vi "Write Case Sensitive Pop-up.vi"(8 "error in (no error)":errorcluster, 10 "CaseSensitivePopup":bool, 11 "ComboBox.lvclass in":refnum<class "ComboBox.lvclass">) -> (0 "error out":errorcluster, 3 "ComboBox.lvclass out":refnum<class "ComboBox.lvclass">)   [LabVIEW 2015, in "ComboBox.lvclass"]
uses:
  ComboBox.lvclass
  ComboBox.lvclass/ComboBox.ctl
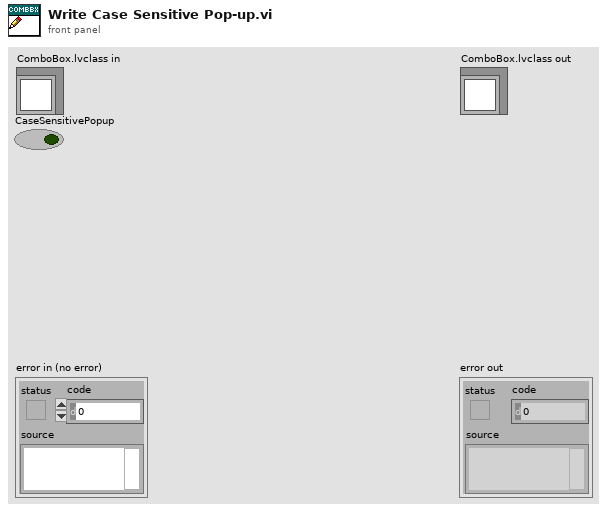
[diagram p1: front panel]
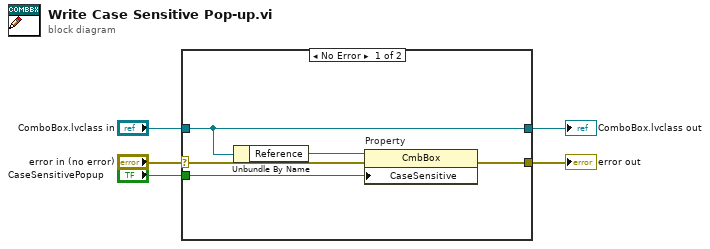
[diagram p0: block diagram]
diagram:
  n1 = case shown="No Error" "error in (no error)" {
    selector: "error in (no error)" -> [w6 w12]
    tunnel: [w10 w12] -> w4
    tunnel: [w8 w11] -> w2
    tunnel: "ComboBox.lvclass in" -> [w8 w11]
    tunnel: "CaseSensitivePopup" -> [w9 _]
    frame No Error {
      n2 = Unbundle By Name(w8) -> ("Reference"=w7:refnum<vi>)
      n3 = property on="Property" class="CmbBox"(reference=w7, error in=w6, "CaseSensitive"=w9) -> (error out=w10:errorcluster)  [unwired: 1 out]
    }
    frame Error {
    }
  }
  "error out" <- w4
  "ComboBox.lvclass out" <- w2
